vi "DHT.vi"() -> ()   [LabVIEW 2018]
uses:
  <vilib>/Utility/file.llb/Write Delimited Spreadsheet (string).vi
  <vilib>/MakerHub/LINX/Public/Utilities/Open Serial.vi
  <vilib>/Utility/file.llb/Write Delimited Spreadsheet (I64).vi
  <vilib>/MakerHub/LINX/LMH-LINX.lvlib
panel:
  out "date/time string":string
  in  "?":enum32{"Temperature", "Humidity"}(tab)
  out "Temperatura":u8(graph)
  out "Umiditate 2":u8(graph)
  out "Humidity %":u8(knob) scale=0.0..100.0
  in  "Serial Port":refnum<visa-resource-name>="N/A"
  out "file or folder exists?":bool
  out "Temp ^C":u8(knob) scale=0.0..50.0
  in  "?":bool
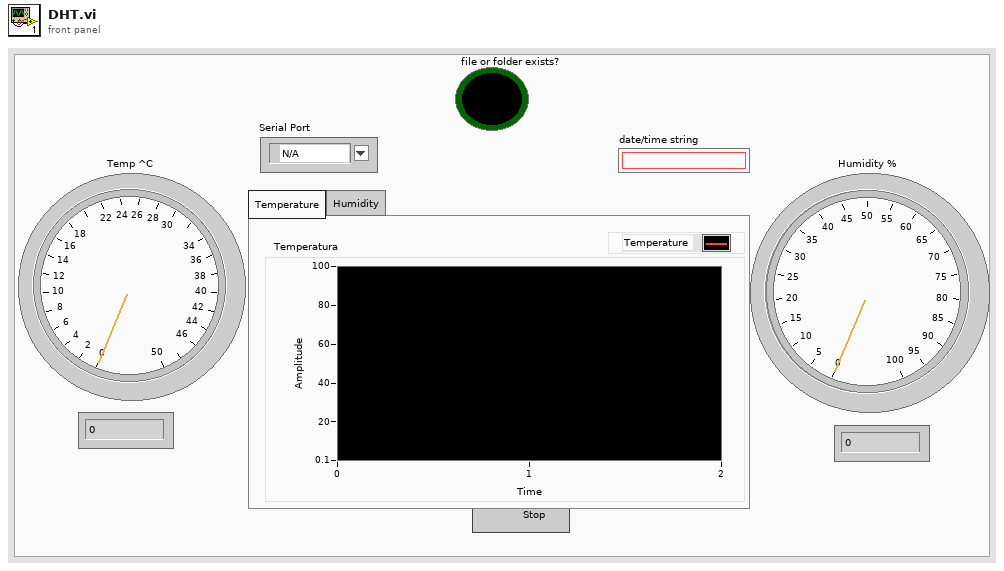
[diagram p1: front panel]
types:
  T1 = enum16{"open", "replace", "create", "open or create", "replace or create", "replace or create with confirmation"}
  T2 = typedef "LMH-LINX.lvlib/LINX Ref.ctl" = cluster{"IO":T3, "Interface":T4, "LINX Device Config":T5}
  T3 = typedef "LMH-LINX.lvlib/Platform.ctl" = enum16{"Remote", "Local"}
  T4 = typedef "LMH-LINX.lvlib/Interface.ctl" = enum16{"Serial", "TCP"}
  T5 = typedef "LMH-LINX.lvlib/Device.lvlib/LINX Device Config.ctl" = cluster{"Interface":T4, "COM Port":refnum<visa-resource-name>, "TCP Configuration":T6, "Device Family":u8, "Device ID":u8, "Device Name":string, "TCP Ref":refnum<k5>, "Channels":T7}
  T6 = typedef "LMH-LINX.lvlib/Device.lvlib/TCP Config.ctl" = cluster{"IP Address":string, "Port":u16}
  T7 = typedef "LMH-LINX.lvlib/Channels.ctl" = cluster{"DI":u8[], "DO":u8[], "AI":u8[], "AO":u8[], "PWM":u8[], "QE":u8[], "UART":u8[], "I2C 2":u8[], "SPI":u8[], "CAN":u8[], "Servo":u8[], "AI Ref (V)":dbl, "AI Resolution (Bits)":u8, "AO Ref (V)":dbl, "AO Resolution (Bits)":u8}
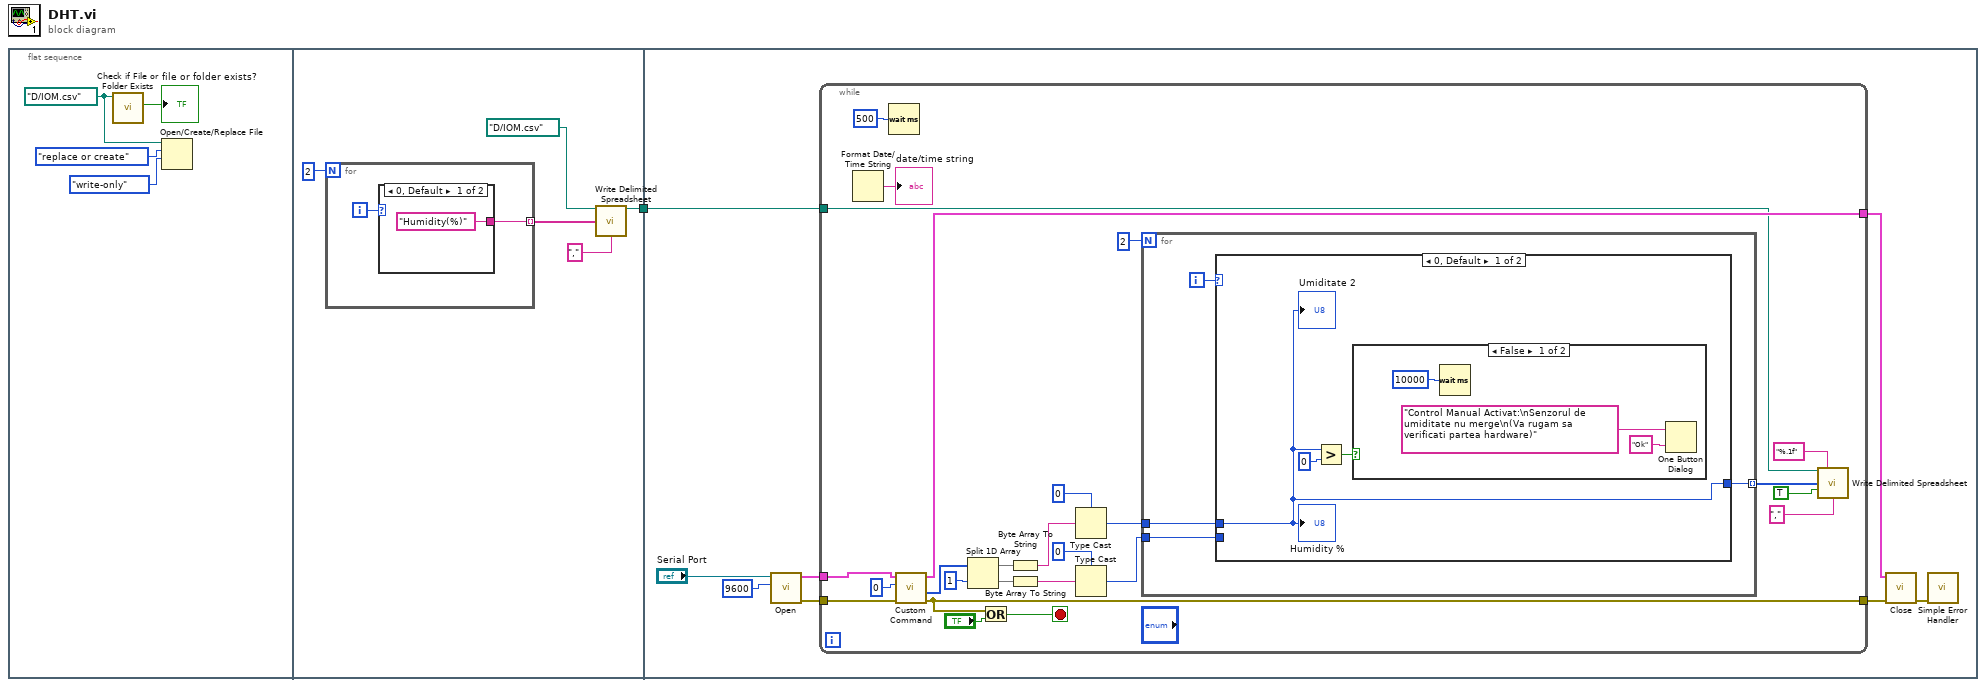
[diagram p0: block diagram]
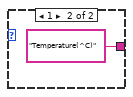
[diagram p2: hidden frame]
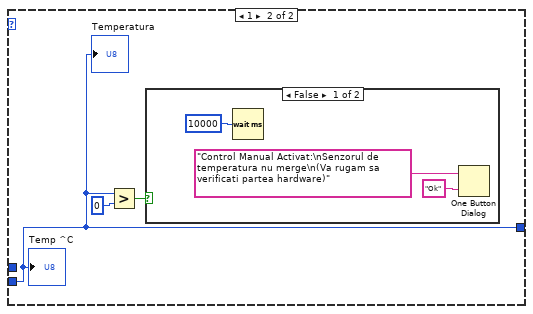
[diagram p4: hidden frame]
diagram:
  n1 = flat-sequence {
    tunnel: [w6] -> w1
    tunnel: w1 -> [w16]
    frame #0 {
      w4 = path "D:/IOM.csv" ("path")
      n2 = call <vilib>:"Check if File or Folder Exists.vi"("path"=w4) -> ("file or folder exists?"=→"file or folder exists?":bool)  [unwired: 8 in, 2 out]
      n3 = Open/Create/Replace File(file path (use dialog)=w4, operation (0:open)=T1."replace or create", access (0:read/write)=enum16{"read/write", "read-only", "write-only"}."write-only") -> ()  [unwired: 3 in, 3 out]
    }
    frame #1 {
      n4 = for {
        N: 2 -> [_]
        tunnel: [w11] -> w7 mode=indexing
        i -> [w12]
        n5 = case shown="0, Default" w12 {
          tunnel: ["Humidity(%)" "Temperature(^C)"] -> w11
          frame 0, Default {
          }
          frame 1 {
          }
        }
      }
      n6 = call-poly <vilib>:"Write Delimited Spreadsheet.vi"("file path (dialog if empty)"=path "D:/IOM.csv", "1D data"=w7, "delimiter (\\t)"="," ("delimiter (\\t)")) -> ("new file path (Not A Path if cancelled)"=w6:path)  [unwired: 11 in, 1 out]
    }
    frame #2 {
      n7 = call-poly <vilib>:"Open.vi"("Baud Rate Override"=u32 9600, "Serial Port"="Serial Port") -> ("Error Out"=w21:errorcluster, "LINX Resource"=w22:T2)  [unwired: 7 in, 1 out]
      n8 = while {
        tunnel: w22 -> [w47]
        tunnel: w21 -> [w46]
        tunnel: [w33] -> w20
        tunnel: [w30] -> w19
        tunnel: w16 -> [w24]
        stop <- w32 stop-if-true
        n9 = Format Date/Time String() -> (date/time string=→"date/time string":string)  [unwired: 3 in]
        n10 = Wait (ms)(milliseconds to wait=u32 500) -> ()  [unwired: 1 out]
        n11 = call <vilib>:"Custom Command.vi"("Error In"=w46, "Custom Command Number"=u16 0, "LINX Resource"=w47) -> ("Error Out"=w30:errorcluster, "Response"=w43:u8[], "LINX Resource"=w33:T2)  [unwired: 5 in, 1 out]
        n12 = Split 1D Array(array=w43, index=1) -> (first subarray=w41:u8[], second subarray=w40:u8[])
        n13 = Or(x=w30, y="?") -> (x .or. y?=w32:bool)
        n14 = Byte Array To String(unsigned byte array=w41) -> (string=w38:string)
        n15 = Byte Array To String(unsigned byte array=w40) -> (string=w36:string)
        n16 = Type Cast(type=u8 0, x=w38) -> (*(type *) &x=w35:u8)
        n17 = Type Cast(type=u8 0, x=w36) -> (*(type *) &x=w34:u8)
        n18 = for {
          N: 2 -> [_]
          tunnel: w35 -> [w50]
          tunnel: w34 -> [w49]
          tunnel: [w48] -> w28 mode=indexing
          i -> [w51]
          n19 = case shown="0, Default" w51 {
            tunnel: w50 -> [w54 _]
            tunnel: w49 -> [_ w59]
            tunnel: [w54 w59] -> w48
            frame 0, Default {
              n20 = Greater?(x=w54, y=u8 0) -> (0:w52:bool)
              n21 = case shown="False" w52 {
                frame False {
                  n22 = Wait (ms)(milliseconds to wait=u32 10000) -> ()  [unwired: 1 out]
                  n23 = One Button Dialog(message="Control Manual Activat:\nSenzorul de umiditate nu merge\n(Va rugam sa verificati partea hardware)", button name ("OK")="Ok") -> ()  [unwired: 1 out]
                }
                frame True {
                }
              }
              "Humidity %" <- w54
              "Umiditate 2" <- w54
            }
            frame 1 {
              n24 = Greater?(x=w59, y=u8 0) -> (0:w58:bool)
              n25 = case shown="False" w58 {
                frame False {
                  n26 = Wait (ms)(milliseconds to wait=u32 10000) -> ()  [unwired: 1 out]
                  n27 = One Button Dialog(message="Control Manual Activat:\nSenzorul de temperatura nu merge\n(Va rugam sa verificati partea hardware)", button name ("OK")="Ok") -> ()  [unwired: 1 out]
                }
                frame True {
                }
              }
              "Temp ^C" <- w59
              "Temperatura" <- w59
            }
          }
        }
        n28 = call-poly <vilib>:"Write Delimited Spreadsheet.vi"("file path (dialog if empty)"=w24, "format (%d)"="%.1f" ("format (%.3f)"), "1D data"=w28, "append to file? (new file:F)"=TRUE, "delimiter (\\t)"="," ("delimiter (\\t)")) -> ()  [unwired: 9 in, 2 out]
      }
      n29 = call <vilib>:"Close.vi"("Error In"=w19, "LINX Resource"=w20) -> ("Error Out"=w15:errorcluster)  [unwired: 9 in]
      n30 = call <vilib>:"Simple Error Handler.vi"("error in (no error)"=w15) -> ()  [unwired: 4 in, 5 out]
    }
  }
